vi "Setup.vi"(10 "Setup":refnum<class "Setup.lvclass">, 11 "Core Actor in":refnum<class "Core Actor.lvclass">) -> (0 "Error out":errorcluster, 3 "Core Actor out":refnum<class "Core Actor.lvclass">)   [LabVIEW 2025, in "jettl.lvlib" / "Core Actor.lvlib" / "Core Actor.lvclass"]
uses:
  Core Actor.lvclass
  Setup/Setup/Setup.lvclass
  Attributes.ctl
  Transport/Transport/Transport.lvclass
  Msg Set.ctl
  Msg/Msg.lvclass
  Core Actor.lvclass/Core Actor.ctl
  Attributes/Attributes.lvlib
  jettl.lvlib
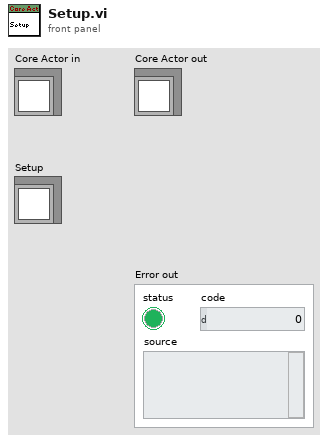
[diagram p1: front panel]
types:
  T1 = typedef "jettl.lvlib/Attributes.ctl" = cluster{"UID":string, "Transport":refnum<class "Transport.lvclass">, "Unified Msg Set":T2, "Actor Ref":refnum<vi>, "Application Ref":refnum<vi>}
  T2 = typedef "jettl.lvlib/Msg Set.ctl" = set{refnum<class "Msg.lvclass">}
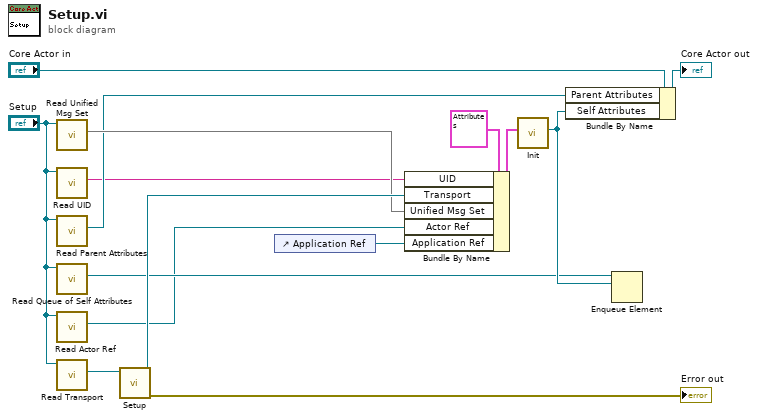
[diagram p0: block diagram]
diagram:
  n1 = call-dynamic "Read Unified Msg Set.vi"("Setup in"="Setup") -> ("Unified Msg Set"=w6:T2)  [unwired: 10 in]
  n2 = call-dynamic "Read UID.vi"("Setup in"="Setup") -> ("UID"=w2:string)  [unwired: 10 in]
  n3 = call-dynamic "Read Parent Attributes.vi"("Setup in"="Setup") -> ("Parent Attributes"=w5:refnum<class "Attributes.lvclass">)  [unwired: 10 in]
  n4 = call-dynamic "Read Queue of Self Attributes.vi"("Setup in"="Setup") -> ("Queue of Self Attributes"=w4:refnum<queue>)  [unwired: 10 in]
  n5 = call-dynamic "Read Actor Ref.vi"("Setup in"="Setup") -> ("Actor Ref"=w3:refnum<vi>)  [unwired: 10 in]
  n6 = call-dynamic "Read Transport.vi"("Setup in"="Setup") -> ("Transport"=w1:refnum<class "Transport.lvclass">)  [unwired: 10 in]
  n7 = call-dynamic "Setup.vi"("Transport in"=w1) -> ("Error out"=→"Error out":errorcluster, "Transport out"=w8:refnum<class "Transport.lvclass">)  [unwired: 9 in]
  n8 = control-ref of="Application Ref"() -> (w11:refnum<vi>)
  n9 = Bundle By Name(cluster=T1 {"UID"="", "Transport"=refnum, "Unified Msg Set"={}, "Actor Ref"=refnum, "Application Ref"=refnum} ("Attributes"), "UID"=w2, "Transport"=w8, "Unified Msg Set"=w6, "Actor Ref"=w3, "Application Ref"=w11) -> (w10:T1)
  n10 = call "Init.vi"("Attributes"=w10) -> ("Attributes"=w13:refnum<class "Attributes.lvclass">)  [unwired: 10 in]
  n11 = Bundle By Name(cluster="Core Actor in", "Parent Attributes"=w5, "Self Attributes"=w13) -> (→"Core Actor out":refnum<class "Core Actor.lvclass">)
  n12 = Enqueue Element(queue=w4, element=w13) -> ()  [unwired: 2 in, 3 out]
